vi "Not A Config Data Refnum.vi"(1 "refnum":T1) -> (0 "not a config data refnum":bool)   [LabVIEW 2010, in "NI_LVConfig.lvlib"]
doc: "Determines whether a configuration data refnum is valid."
uses:
  NI_LVConfig.lvlib
  Config Data RefNum.ctl
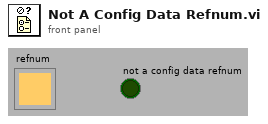
[diagram p1: front panel]
types:
  T1 = typedef "NI_LVConfig.lvlib/Config Data RefNum.ctl" = refnum<k1>
  T2 = typedef "NI_LVConfig.lvlib/Config Queue.ctl" = refnum<queue>
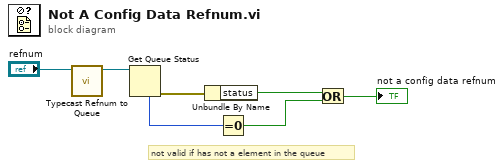
[diagram p0: block diagram]
diagram:
  # "not valid if has not a element in the queue"
  n1 = call "Typecast Refnum to Queue.vi"("refnum in"="refnum") -> ("queue out"=w7:T2)  [unwired: 10 in]
  n2 = Get Queue Status(queue=w7) -> (error out=w4:errorcluster, # elements in queue=w6:i32)  [unwired: 1 in, 7 out]
  n3 = Unbundle By Name(w4) -> ("status"=w3:bool)
  n4 = Equal To 0?(x=w6) -> (x = 0?=w2:bool)
  n5 = Or(x=w3, y=w2) -> (x .or. y?=→"not a config data refnum":bool)
